vi "Step_electromagnet.vi"(0 "VISA Refnum in":refnum<visa-resource-name>, 1 "Up/dn in":bool, 5 "Actual Voltage (V)":dbl, 9 "Min Voltage (V) in":dbl, 11 "error in (no error)":errorcluster, 12 "Max Voltage (V)":dbl, 13 "Voltage Step (V)":dbl) -> (4 "Up/dn out":bool, 6 "Min Voltage (V) out":dbl, 15 "error out":errorcluster)   [LabVIEW 2017]
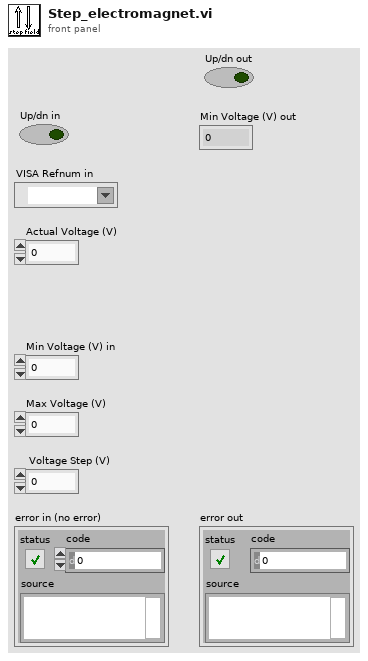
[diagram p1: front panel]
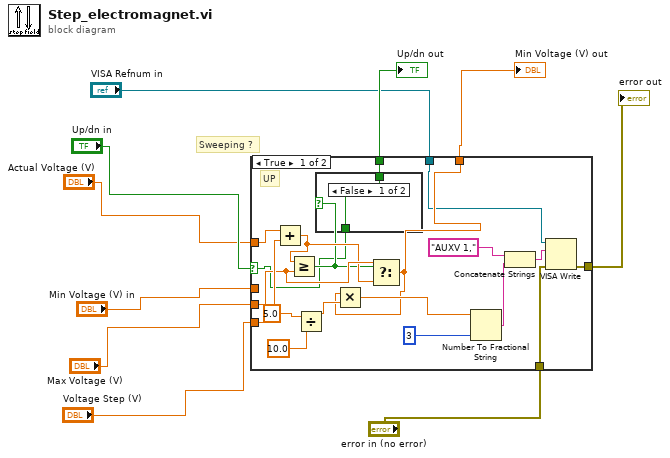
[diagram p0: block diagram]
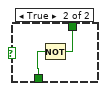
[diagram p2: hidden frame]
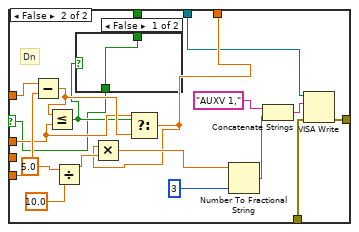
[diagram p3: hidden frame]
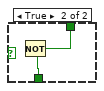
[diagram p4: hidden frame]
diagram:
  # "Sweeping ?"
  n1 = case shown="True" "Up/dn in" {
    selector: "Up/dn in" -> [w14 w36]
    tunnel: "Actual Voltage (V)" -> [w29 w51]
    tunnel: "Max Voltage (V)" -> [w27 _]
    tunnel: "Voltage Step (V)" -> [w28 w50]
    tunnel: [w18 w41] -> w6
    tunnel: "error in (no error)" -> [w17 w40]
    tunnel: "Min Voltage (V) in" -> [_ w38]
    tunnel: [w13 w35] -> w8
    tunnel: "VISA Refnum in" -> [w12 w34]
    tunnel: [w11 w33] -> w10
    frame True {
      # "UP"
      n2 = Add(x=w29, y=w28) -> (x+y=w26:dbl)
      n3 = Greater Or Equal?(x=w26, y=w27) -> (x >= y?=w15:bool)
      n4 = Divide(x=5.0 ("y"), y=10.0) -> (x/y=w21:dbl)
      n5 = case shown="False" w15 {
        tunnel: w14 -> [w30 w32]
        tunnel: [w30 w31] -> w11
        frame False {
        }
        frame True {
          n6 = Not(x=w32) -> (.not. x?=w31:bool)
        }
      }
      n7 = Select(t=w27, s=w15, f=w26) -> (s? t:f=w13:dbl)
      n8 = Multiply(x=w13, y=w21) -> (x*y=w16:dbl)
      n9 = Number To Fractional String(number=w16, precision (6)=i16 3) -> (F-format string=w23:string)  [unwired: 2 in]
      n10 = Concatenate Strings("AUXV 1," ("data"), w23) -> (w25:string)
      n11 = VISA Write(VISA resource name=w12, write buffer=w25, error in (no error)=w17) -> (error out=w18:errorcluster)  [unwired: 2 out]
    }
    frame False {
      # "Dn"
      n12 = Subtract(x=w51, y=w50) -> (x-y=w49:dbl)
      n13 = Less Or Equal?(x=w49, y=w38) -> (x <= y?=w37:bool)
      n14 = Divide(x=5.0 ("y"), y=10.0) -> (x/y=w44:dbl)
      n15 = case shown="False" w37 {
        tunnel: w36 -> [w52 w54]
        tunnel: [w52 w53] -> w33
        frame False {
        }
        frame True {
          n16 = Not(x=w54) -> (.not. x?=w53:bool)
        }
      }
      n17 = Select(t=w38, s=w37, f=w49) -> (s? t:f=w35:dbl)
      n18 = Multiply(x=w35, y=w44) -> (x*y=w39:dbl)
      n19 = Number To Fractional String(number=w39, precision (6)=i16 3) -> (F-format string=w46:string)  [unwired: 2 in]
      n20 = Concatenate Strings("AUXV 1," ("data"), w46) -> (w48:string)
      n21 = VISA Write(VISA resource name=w34, write buffer=w48, error in (no error)=w40) -> (error out=w41:errorcluster)  [unwired: 2 out]
    }
  }
  "Up/dn out" <- w10
  "Min Voltage (V) out" <- w8
  "error out" <- w6
